vi "Pedestrian Signal Controller.vi"(11 "cars stopped":T1) -> (0 "ped signal":T2, 3 "peds stopped":T1)   [LabVIEW 2023]
uses:
  <extravilib>/ChannelInstances/One Element Stream-u16/)Channel.ctl
  <extravilib>/ChannelInstances/One Element Stream-bool/)Channel.ctl
  b437e94f-365f-2543-b817-94f850b61798.vi
  091f0f9f-ba83-5e49-bf52-7e477d967a4d.vi
  <extravilib>/ChannelInstances/One Element Stream-u16/Write With Abort.vi
  <extravilib>/ChannelInstances/One Element Stream-bool/Write With Abort.vi
  <extravilib>/ChannelInstances/One Element Stream-bool/Read With Abort.vi
  <extravilib>/ChannelInstances/One Element Stream-u16/Endpoint.vi
  <extravilib>/ChannelInstances/One Element Stream-bool/Endpoint.vi
  <extravilib>/ChannelInstances/One Element Stream-bool/EndpointRead.vi
  <extravilib>/ChannelInstances/One Element Stream-bool.lvlib
  <extravilib>/ChannelInstances/One Element Stream-u16.lvlib
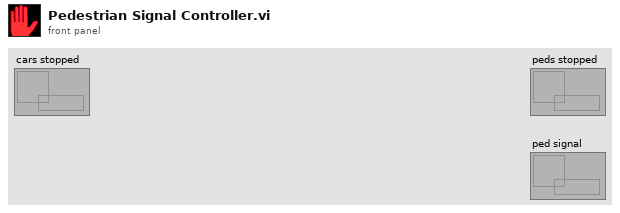
[diagram p1: front panel]
types:
  T1 = typedef "One Element Stream-bool.lvlib/)Channel.ctl" = refnum<queue>
  T2 = typedef "One Element Stream-u16.lvlib/)Channel.ctl" = refnum<queue>
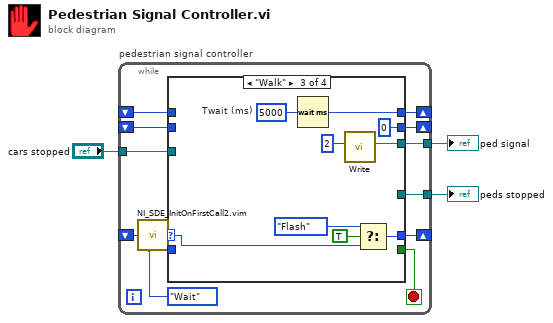
[diagram p0: block diagram]
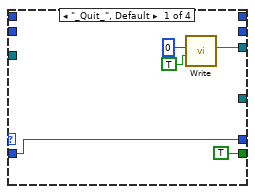
[diagram p2: hidden frame]
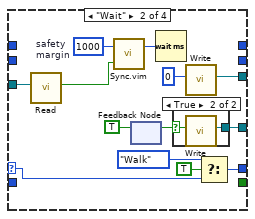
[diagram p3: hidden frame]
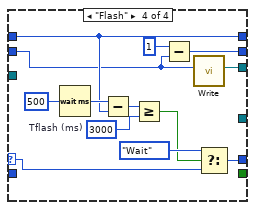
[diagram p5: hidden frame]
diagram:
  n1 = while "pedestrian signal controller" {
    tunnel: "cars stopped" -> [w14]
    shift-right: [w13] -> _
    shift-left: _ -> [w12]
    tunnel: [w11] -> w3
    shift-right: [w10] -> _
    shift-left: _ -> [w9]
    tunnel: [w8] -> w2
    shift-right: [w5] -> _
    shift-left: _ -> [w6]
    stop <- w15 stop-if-true
    w7 = enum16{"_Quit_", "Wait", "Walk", "Flash"}."Wait"
    n2 = call "NI_SDE_InitOnFirstCall2.vim"("input"=w6, "master enum"=w7) -> ("output enum"=w4:enum16{"_Quit_", "Wait", "Walk", "Flash"})  [unwired: 1 in]
    n3 = case shown="\"Walk\"" w4 {
      selector: w4 -> [_ w33 w44 w57]
      tunnel: [TRUE _ _ _] -> w15
      tunnel: [w16 w32 w43 w56] -> w5
      tunnel: w14 -> [_ w30 _ _]
      tunnel: [_ _ w39 w50] -> w13
      tunnel: w12 -> [_ _ _ w50]
      tunnel: [w18 w28 w37 w49] -> w11
      tunnel: [_ _ u16 0 w47] -> w10
      tunnel: w9 -> [_ _ _ w46]
      tunnel: [_ w27 _ _] -> w8
      tunnel: w7 -> [w16 _ _ _]
      frame "_Quit_", Default {
        n4 = call <extravilib>:"Write.vi"("last element? (F)"=TRUE, "element"=u16 0) -> ("channel"=w18:T2)  [unwired: 8 in, 1 out]
      }
      frame "Wait" {
        w24 = u32 1000  # safety margin
        n5 = call <extravilib>:"Read.vi"("channel"=w30) -> ("element"=w25:bool)  [unwired: 7 in, 3 out]
        n6 = call "Sync.vim"("a"=w24, "b"=w25) -> ("a'"=w23:u32)  [unwired: 24 in, 1 out]
        n7 = feedback-in #1(TRUE) -> ()
        n8 = feedback #1() -> (w21:bool)  [unwired: 1 in]
        n9 = Wait (ms)(milliseconds to wait=w23) -> ()  [unwired: 1 out]
        n10 = case shown="True" w21 {
          selector: w21 -> [_ w34]
          tunnel: [_ w35] -> w27
          frame False {
          }
          frame True {
            n11 = call <extravilib>:"Write.vi"("element"=w34) -> ("channel"=w35:T1)  [unwired: 9 in, 1 out]
          }
        }
        n12 = call <extravilib>:"Write.vi"("element"=u16 0) -> ("channel"=w28:T2)  [unwired: 9 in, 1 out]
        n13 = Select(t=enum16{"_Quit_", "Wait", "Walk", "Flash"}."Walk", s=TRUE, f=w33) -> (s? t:f=w32:enum16{"_Quit_", "Wait", "Walk", "Flash"})
      }
      frame "Walk" {
        w41 = u32 5000  # Twait (ms)
        n14 = Wait (ms)(milliseconds to wait=w41) -> (millisecond timer value=w39:u32)
        n15 = call <extravilib>:"Write.vi"("element"=u16 2) -> ("channel"=w37:T2)  [unwired: 9 in, 1 out]
        n16 = Select(t=enum16{"_Quit_", "Wait", "Walk", "Flash"}."Flash", s=TRUE, f=w44) -> (s? t:f=w43:enum16{"_Quit_", "Wait", "Walk", "Flash"})
      }
      frame "Flash" {
        w51 = u32 3000  # Tflash (ms)
        n17 = Wait (ms)(milliseconds to wait=u32 500) -> (millisecond timer value=w53:u32)
        n18 = Subtract(x=w53, y=w50) -> (x-y=w52:u32)
        n19 = Greater Or Equal?(x=w52, y=w51) -> (x >= y?=w45:bool)
        n20 = Subtract(x=u16 1, y=w46) -> (x-y=w47:u16)
        n21 = call <extravilib>:"Write.vi"("element"=w46) -> ("channel"=w49:T2)  [unwired: 9 in, 1 out]
        n22 = Select(t=enum16{"_Quit_", "Wait", "Walk", "Flash"}."Wait", s=w45, f=w57) -> (s? t:f=w56:enum16{"_Quit_", "Wait", "Walk", "Flash"})
      }
    }
  }
  "ped signal" <- w3
  "peds stopped" <- w2
